vi "Setup.vi"(8 "error in (no error)":errorcluster, 11 "Configuration File Interface Test In":refnum<class "Configuration File Process Interface Test.lvclass">) -> (0 "error out":errorcluster, 3 "Configuration File Interface Test Out":refnum<class "Configuration File Process Interface Test.lvclass">)   [LabVIEW 2020, in "Configuration File Process Interface Test.lvclass"]
uses:
  Configuration File Process Interface Test.lvclass
  Configuration File Process Interface Test.lvclass/Configuration File Process Interface Test.ctl
  Configuration Interface Test/Configuration Interface Test.lvclass
  Mock Configurable Process/Mock Configurable Process.lvclass
  C:/Git/triarc-framework/source/Framework/Process/Process.lvclass
  C:/Git/triarc-framework/source/Framework/Base/Base.lvclass
  C:/Git/triarc-framework/source/Framework/Configuration File/Configuration File.lvclass
  C:/Git/triarc-framework/source/Framework/Configuration/Configuration.lvclass
  C:/Git/triarc-framework/source/Framework/Error Handler Interface/Error Handler Interface.lvclass
  C:/Git/triarc-framework/source/Framework/Logging/Logging.lvclass
  C:/Git/triarc-framework/source/Framework Test/Mock Configurable Process/Mock Configurable Process.lvclass
  C:/Git/triarc-framework/source/Framework Test/Configuration Interface Test/Configuration Interface Test.lvclass
  C:/Program Files (x86)/National Instruments/LabVIEW 2020/vi.lib/Astemes/LUnit/Test Case.lvclass
  C:/Git/triarc-framework/source/Framework Test/Configuration File Process Interface Test/Configuration File Process Interface Test.lvclass
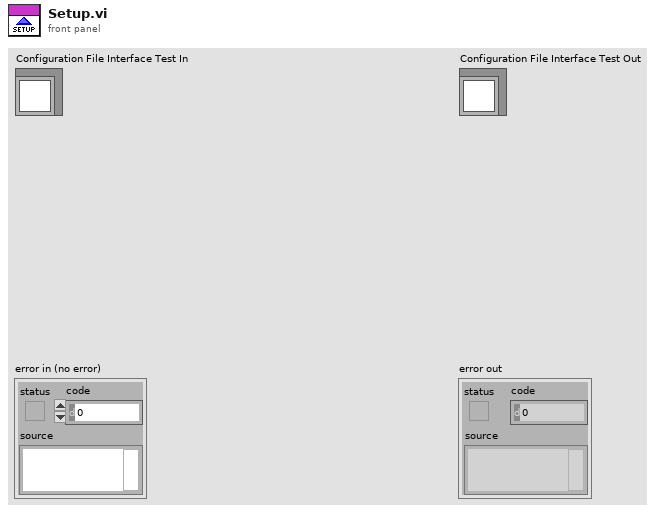
[diagram p1: front panel]
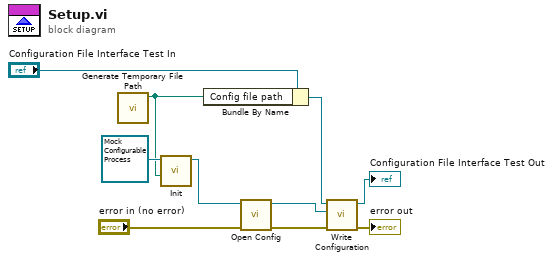
[diagram p0: block diagram]
diagram:
  n1 = call <vilib>:"Generate Temporary File Path.vi"() -> ("Unique Temporary File Path"=w1:path)  [unwired: 10 in, 1 out]
  n2 = call-dynamic "Init.vi"("Config File Path"=w1, "Process In"=refnum<class "Mock Configurable Process.lvclass"> refnum ("Mock Configurable.lvclass")) -> ("Process Out"=w3:refnum<class "Mock Configurable Process.lvclass">)  [unwired: 8 in, 1 out]
  n3 = Bundle By Name(cluster="Configuration File Interface Test In", "Config file path"=w1) -> (w2:refnum<class "Configuration File Process Interface Test.lvclass">)
  n4 = call-dynamic "Open Config.vi"("error in (no error)"="error in (no error)", "Configuration File File In"=w3) -> ("error out"=w4:errorcluster, "Configuration File File Out"=w6:refnum<class "Mock Configurable Process.lvclass">)  [unwired: 8 in]
  n5 = call "Write Configuration.vi"("error in (no error)"=w4, "Configuration"=w6, "Configuration Interface Test In"=w2) -> ("error out"=→"error out":errorcluster, "Configuration Interface Test Out"=→"Configuration File Interface Test Out":refnum<class "Configuration File Process Interface Test.lvclass">)  [unwired: 7 in]
